vi "HEI_Data_single.vi"(0 "params":dbl[](array[numeric])) -> (8 "RPM":dbl, 9 "Dynamic Data":dynamicdata(waveform), 10 "RPM 2":dbl format="RPM:          %#_g", 13 "Torque 2":dbl format="Torque:      %#_g", 14 "Waveform Chart 4":dynamicdata(graph), 16 "Torque":dbl, 18 "Waveform Chart 6":dynamicdata(graph))   [LabVIEW 2017]
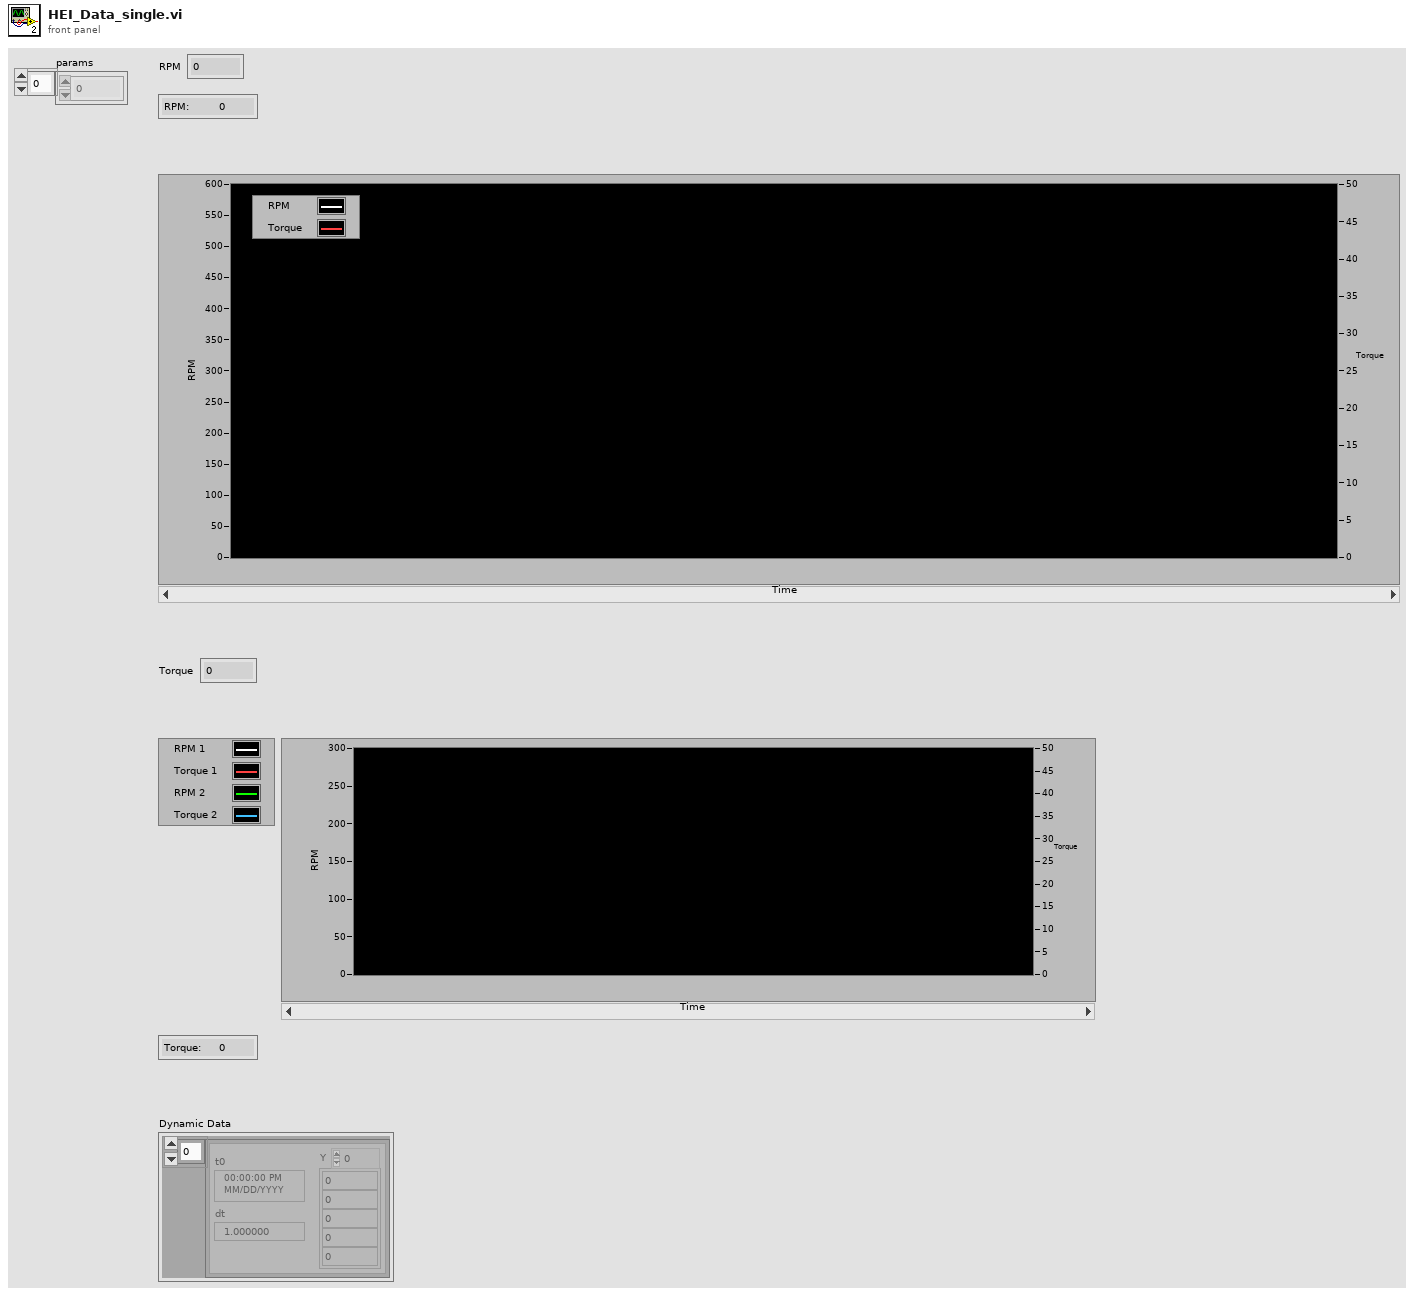
[diagram p1: front panel]
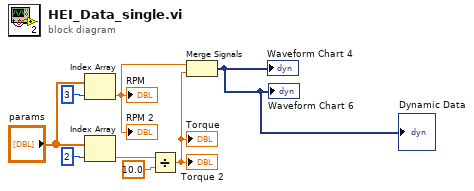
[diagram p0: block diagram]
diagram:
  n1 = Index Array(array="params", index=3) -> (element=w6:dbl)
  "RPM" <- w6
  "RPM 2" <- w6
  n2 = Index Array(array="params", index=2) -> (element=w4:dbl)
  n3 = Divide(x=w4, y=10.0) -> (x/y=w7:dbl)
  "Torque" <- w7
  "Torque 2" <- w7
  n4 = Merge Signals(w6, w7) -> (→"Waveform Chart 4" →"Waveform Chart 6" →"Dynamic Data":dynamicdata)
